vi "boardinfo.vi"(1 "VCI_BOARD_INFO":T1) -> ()   [LabVIEW 2017]
panel:
  out "VCI_BOARD_INFO 2":T1
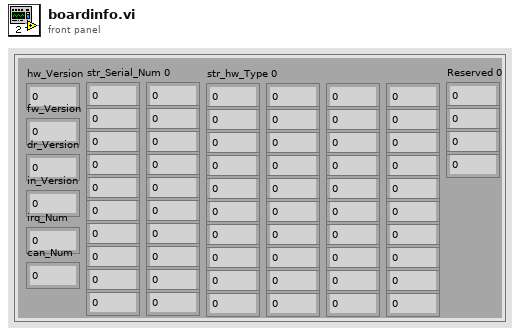
[diagram p1: front panel]
types:
  T1 = cluster{"hw_Version":u16, "fw_Version":u16, "dr_Version":u16, "in_Version":u16, "irq_Num":u16, "can_Num":u8, "str_Serial_Num 0":i8, "str_Serial_Num 1":i8, "str_Serial_Num 2":i8, "str_Serial_Num 3":i8, "str_Serial_Num 4":i8, "str_Serial_Num 5":i8, "str_Serial_Num 6":i8, "str_Serial_Num 7":i8, "str_Serial_Num 8":i8, "str_Serial_Num 9":i8, "str_Serial_Num 10":i8, "str_Serial_Num 11":i8, "str_Serial_Num 12":i8, "str_Serial_Num 13":i8, "str_Serial_Num 14":i8, "str_Serial_Num 15":i8, "str_Serial_Num 16":i8, "str_Serial_Num 17":i8, "str_Serial_Num 18":i8, "str_Serial_Num 19":i8, "str_hw_Type 0":i8, "str_hw_Type 1":i8, "str_hw_Type 2":i8, "str_hw_Type 3":i8, "str_hw_Type 4":i8, "str_hw_Type 5":i8, "str_hw_Type 6":i8, "str_hw_Type 7":i8, "str_hw_Type 8":i8, "str_hw_Type 9":i8, "str_hw_Type 10":i8, "str_hw_Type 11":i8, "str_hw_Type 12":i8, "str_hw_Type 13":i8, "str_hw_Type 14":i8, "str_hw_Type 15":i8, "str_hw_Type 16":i8, "str_hw_Type 17":i8, "str_hw_Type 18":i8, "str_hw_Type 19":i8, "str_hw_Type 20":i8, "str_hw_Type 21":i8, "str_hw_Type 22":i8, "str_hw_Type 23":i8, "str_hw_Type 24":i8, "str_hw_Type 25":i8, "str_hw_Type 26":i8, "str_hw_Type 27":i8, "str_hw_Type 28":i8, "str_hw_Type 29":i8, "str_hw_Type 30":i8, "str_hw_Type 31":i8, "str_hw_Type 32":i8, "str_hw_Type 33":i8, "str_hw_Type 34":i8, "str_hw_Type 35":i8, "str_hw_Type 36":i8, "str_hw_Type 37":i8, "str_hw_Type 38":i8, "str_hw_Type 39":i8, "Reserved 0":u16, "Reserved 1":u16, "Reserved 2":u16, "Reserved 3":u16}
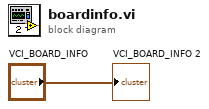
[diagram p0: block diagram]
diagram:
  "VCI_BOARD_INFO 2" <- "VCI_BOARD_INFO"
